vi "Wavenames and comments.vi"(0 "Path":path) -> (1 "Array":string[](array[string]), 2 "Notes":string)   [LabVIEW 2016]
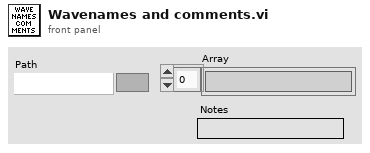
[diagram p1: front panel]
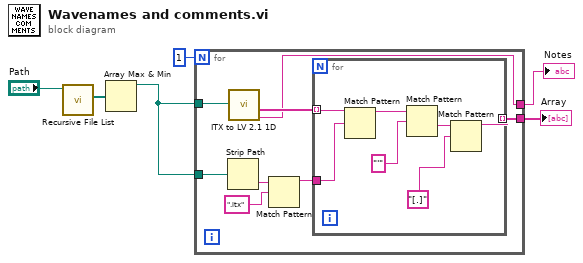
[diagram p0: block diagram]
diagram:
  n1 = call <vilib>:"Recursive File List.vi"("Folder Path"="Path") -> ("All Files in Dir"=w5:path[])  [unwired: 6 in, 4 out]
  n2 = Array Max & Min(array=w5) -> (max value=w2:path)  [unwired: 3 out]
  n3 = for {
    N: 1 -> [_]
    tunnel: w2 -> [w14]
    tunnel: [w13] -> w3
    tunnel: w2 -> [w9]
    tunnel: [w7] -> w1
    n4 = Strip Path(path=w9) -> (name=w10:string)  [unwired: 1 out]
    n5 = call <userlib>:"ITX to LV 2.1 1D.vi"("file (use dialog)"=w14) -> ("wave names"=w12:string[], "Notes"=w7:string)  [unwired: 2 in, 1 out]
    n6 = Match Pattern(string=w10, regular expression=".itx") -> (before substring=w8:string)  [unwired: 1 in, 3 out]
    n7 = for {
      tunnel: [w17] -> w13 mode=indexing
      tunnel: w12 -> [w16] mode=indexing
      tunnel: w8 -> [w15]
      n8 = Match Pattern(string=w16, regular expression=w15) -> (before substring=w20:string)  [unwired: 1 in, 3 out]
      n9 = Match Pattern(string=w20, regular expression="'") -> (after substring=w18:string)  [unwired: 1 in, 3 out]
      n10 = Match Pattern(string=w18, regular expression="[.]") -> (before substring=w17:string)  [unwired: 1 in, 3 out]
    }
  }
  "Array" <- w3
  "Notes" <- w1
